vi "Pre-Build Action.vi"(6 "Top Level/Always Included VIs":path[](array[path]), 7 "Main Destination Path":path, 9 "Target Name":string, 10 "Build Specification Name":string, 11 "Project Path":path) -> (0 "error out":errorcluster)   [LabVIEW 2019]
panel:
  out "ProjectItems":cluster{"Path":path, "Display Name":string}[](array[cluster])
  out "appended path":path
  in  "error in (no error)":errorcluster
  out "error out 2":errorcluster
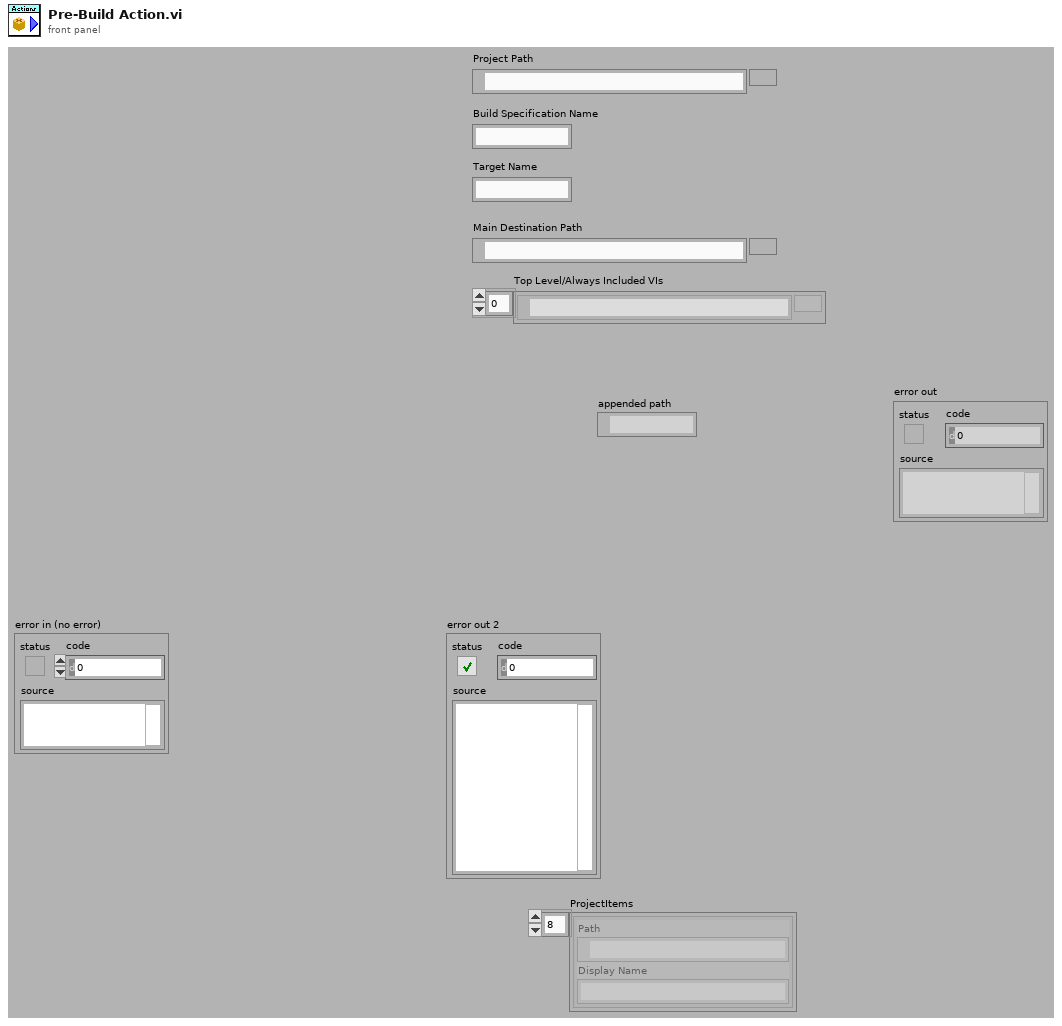
[diagram p1: front panel]
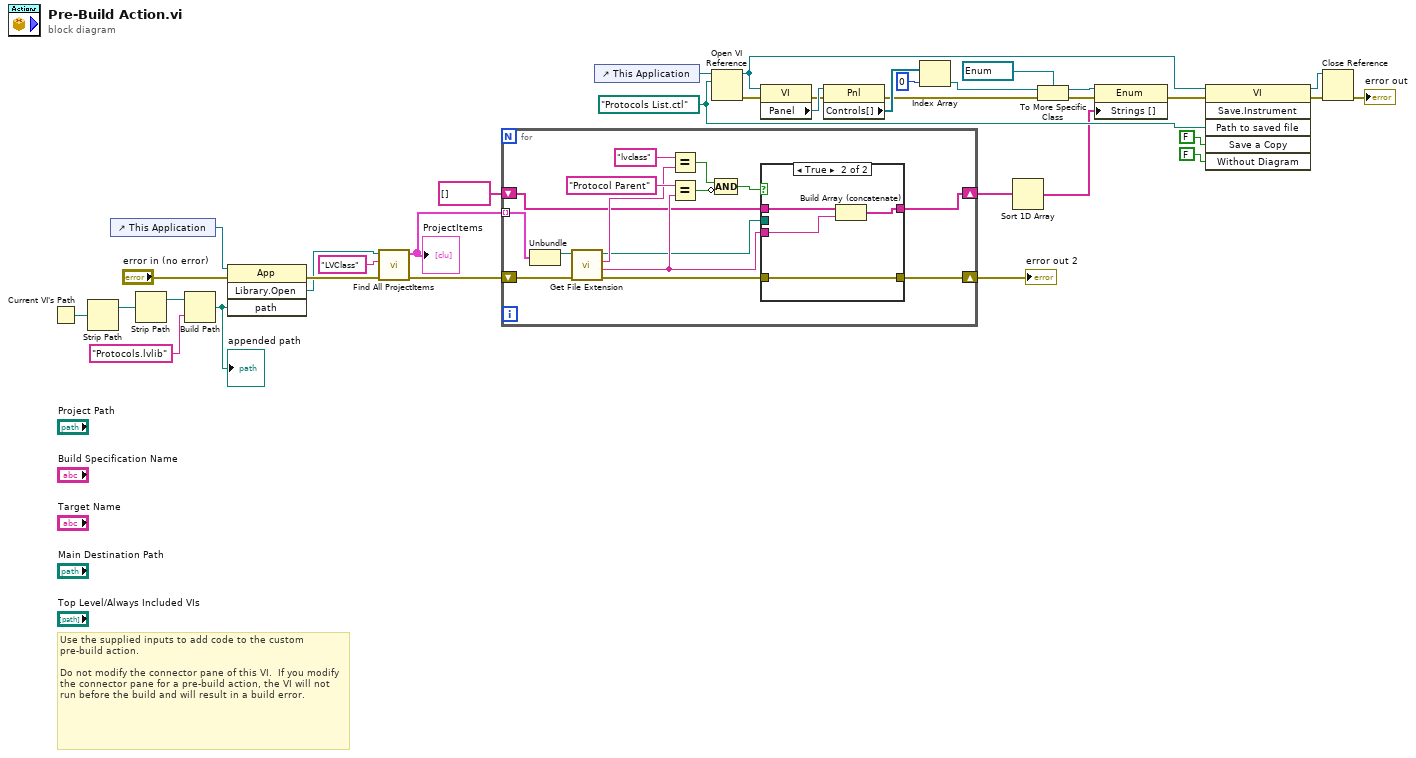
[diagram p0: block diagram]
diagram:
  w28 = path "Protocols List.ctl" ("vi path")
  # "Use the supplied inputs to add code to the custom pre-build action.\n\nDo not modify the connector pane of this VI.  If you modify the connector pane for a pre-build action, the VI will not run before the build and will result in a build error."
  n1 = Current VI's Path() -> (path=w16:path)
  n2 = Strip Path(path=w16) -> (stripped path=w14:path)  [unwired: 1 out]
  n3 = control-ref of="This Application"() -> (w12:refnum<vi>)
  n4 = Strip Path(path=w14) -> (stripped path=w13:path)  [unwired: 1 out]
  n5 = Build Path(base path=w13, name or relative path="Protocols.lvlib") -> (appended path=w10:path)
  "appended path" <- w10
  n6 = invoke class="App" method="Library.Open"(reference=w12, error in="error in (no error)", "path"=w10) -> (error out=w9:errorcluster, "Open Library"=w8:refnum<vi>)  [unwired: 1 in, 2 out]
  n7 = call "Find All ProjectItems.vi"("error in"=w9, "ProjectItem type"="LVClass", "ProjectItem refnum"=w8) -> ("error out"=w7:errorcluster, "ProjectItems"=w4:cluster{"Path":path, "Display Name":string}[])  [unwired: 7 in]
  "ProjectItems" <- w4
  n8 = for {
    shift-right: [w41] -> w5
    shift-left: w7 -> [w46]
    tunnel: w4 -> [w39] mode=indexing
    shift-right: [w36] -> w2
    shift-left: string[] [] -> [w37]
    n9 = Unbundle(w39) -> ("Path"=w38:path)  [unwired: 1 out]
    n10 = call <vilib>:"Get File Extension.vi"("error in (no error)"=w46, "file"=w38) -> ("error out"=w42:errorcluster, "filename without extension"=w44:string, "lowercase file extension"=w47:string, "dup file"=w43:path)  [unwired: 5 in, 1 out]
    n11 = Equal?(x="lvclass" ("string"), y=w47) -> (x = y?=w49:bool)
    n12 = Equal?(x="Protocol Parent", y=w44) -> (x = y?=w45:bool)
    n13 = Compound Arithmetic op=AND(w49, invert w45) -> (w40:bool)
    n14 = case shown="True" w40 {
      tunnel: w44 -> [_ w54]
      tunnel: w43 -> [_ _]
      tunnel: w42 -> [w52 w53]
      tunnel: [w52 w53] -> w41
      tunnel: w37 -> [w51 w56]
      tunnel: [w51 w55] -> w36
      frame False {
      }
      frame True {
        n15 = Build Array (concatenate)(w56, w54) -> (w55:string[])
      }
    }
  }
  "error out 2" <- w5
  n16 = control-ref of="This Application"() -> (w35:refnum<vi>)
  n17 = Open VI Reference(application reference (local)=w35, vi path=w28) -> (vi reference=w29:refnum<vi>, error out=w20:errorcluster)  [unwired: 4 in]
  n18 = property class="VI"(reference=w29, error in=w20) -> (error out=w21:errorcluster, "Panel"=w22:refnum<vi>)  [unwired: 1 out]
  n19 = property class="Pnl"(reference=w22, error in=w21) -> (error out=w23:errorcluster, "Controls[]"=w34:refnum<vi>[])  [unwired: 1 out]
  n20 = Index Array(array=w34, index=0) -> (element=w32:refnum<vi>)
  n21 = Sort 1D Array(array=w2) -> (sorted array=w1:string[])
  n22 = To More Specific Class(target class=refnum<vi> refnum ("reference"), reference=w32, error in=w23) -> (specific class reference=w30:refnum<vi>, error out=w24:errorcluster)
  n23 = property on="Property Node" class="Enum"(reference=w30, error in=w24, "Strings []"=w1) -> (error out=w25:errorcluster)  [unwired: 1 out]
  n24 = invoke class="VI" method="Save.Instrument"(reference=w29, error in=w25, "Path to saved file"=w28, "Save a Copy"=FALSE, "Without Diagram"=FALSE) -> (reference out=w19:refnum<vi>, error out=w18:errorcluster)  [unwired: 1 in, 4 out]
  n25 = Close Reference(reference=w19, error in (no error)=w18) -> (error out=→"error out":errorcluster)
